vi "Read Test Suites.vi"(8 "error in (no error)":errorcluster, 11 "Test Suite In":refnum<class "LUnit Test Suite.lvclass">) -> (0 "error out":errorcluster, 2 "Test Suites":refnum<class "LUnit Test Suite.lvclass">[](array[class]), 3 "Test Suite Out":refnum<class "LUnit Test Suite.lvclass">)   [LabVIEW 2020, in "LUnit Test Suite.lvclass"]
doc: "Get all nested Test Suites."
uses:
  LUnit Test Suite.lvclass
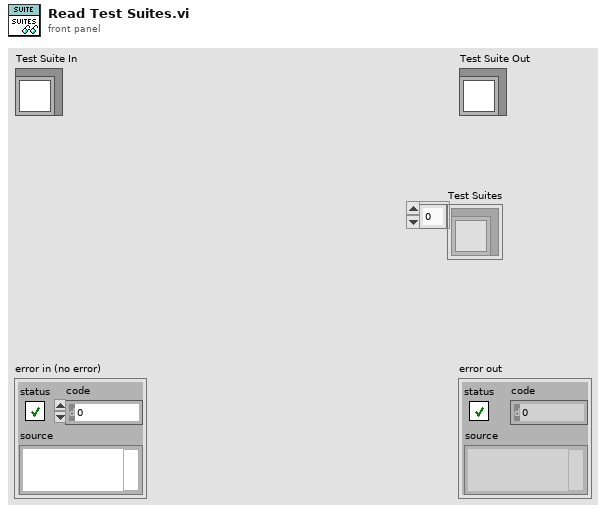
[diagram p1: front panel]
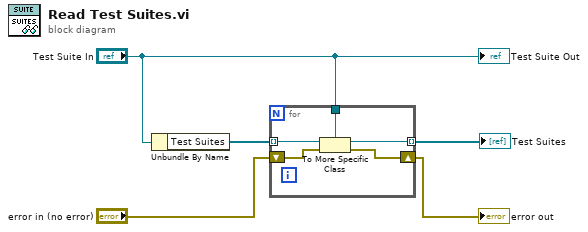
[diagram p0: block diagram]
diagram:
  n1 = Unbundle By Name("Test Suite In") -> ("Test Suites"=w5:refnum<class>[])
  n2 = for {
    tunnel: w5 -> [w10] mode=indexing
    tunnel: "Test Suite In" -> [w9]
    tunnel: [w8] -> w3 mode=indexing
    shift-right: [w6] -> w1
    shift-left: "error in (no error)" -> [w7]
    n3 = To More Specific Class(target class=w9, reference=w10, error in=w7) -> (specific class reference=w8:refnum<class "LUnit Test Suite.lvclass">, error out=w6:errorcluster)
  }
  "error out" <- w1
  "Test Suites" <- w3
  "Test Suite Out" <- "Test Suite In"
